vi "Write Result.vi"(8 "error in (no error)":errorcluster, 11 "TestData":T1 {"data"."Settings"."Source V" format="%#_g V"; "data"."Settings"."VLED 3" format="%#_g V"; "data"."Settings"."VLED 2" format="%#_g V"; "data"."Settings"."VLED 1" format="%#f V"; "data"."Limits"."Wavelength" format="%#_g nm"; "data"."Limits"."Tolerance" format="%#_g %"; "data"."Limits"."Current 3" format="%#_g  mA"; "data"."Limits"."Current 2" format="%#_g  mA"; "data"."Limits"."Current 1" format="%#_g mA"; "data"."Instruments"."Resistor 3" format="%#_g ohm"; "data"."Instruments"."Resistor 2" format="%#_g ohm"; "data"."Instruments"."Resistor 1" format="%#f ohm"}) -> (0 "error out":errorcluster, 2 "History Data":string[](array[string]))   [LabVIEW 2018, in "LED Control Module.lvlib"]
doc: "Very simple result logger - this is a placeholder."
uses:
  LED Control Module.lvlib
  Public Controls/TestData.ctl
  INI/INI File Control.ctl
  Public Controls/LVS Testplan.ctl
  Public Controls/LVS Instruments.ctl
  Public Controls/LVS Limits.ctl
  Public Controls/LVS Settings.ctl
  <vilib>/Utility/file.llb/Write Delimited Spreadsheet (string).vi
  INI/LED INI File.lvlib
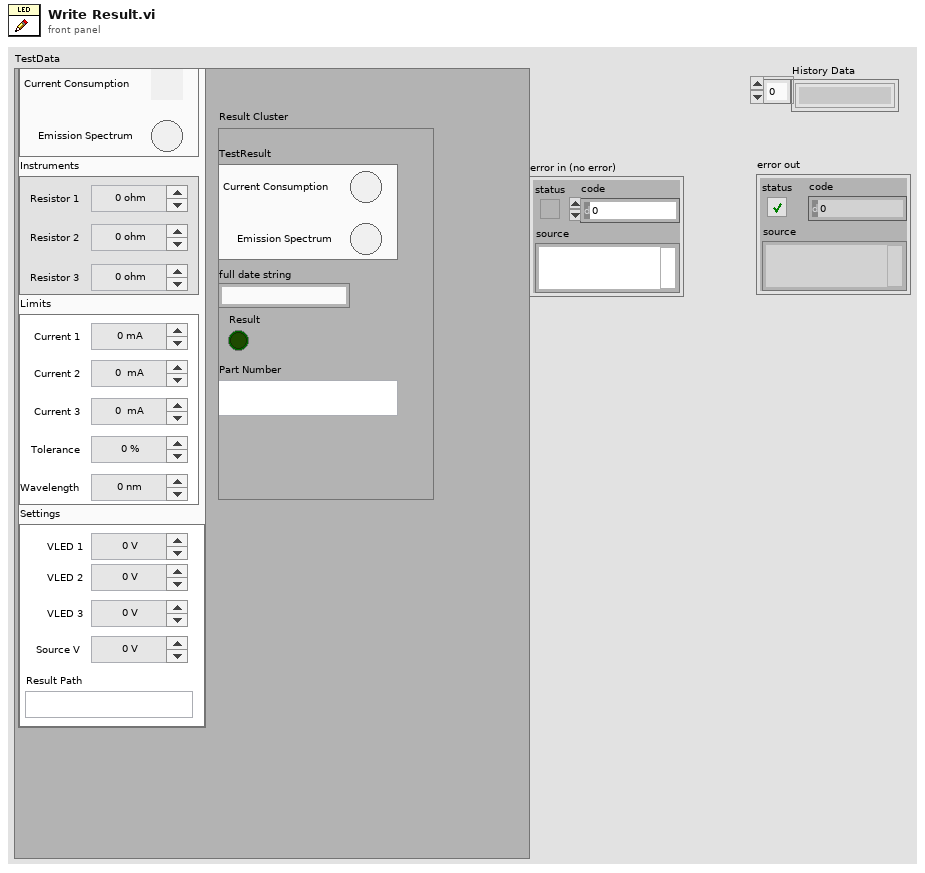
[diagram p1: front panel]
types:
  T1 = typedef "LED Control Module.lvlib/TestData.ctl" = cluster{"data":T2, "Result Cluster":cluster{"TestResult":T3, "full date string":string, "Result":bool, "Part Number":string}}
  T2 = typedef "LED Control Module.lvlib/LED INI File.lvlib/INI File Control.ctl" = cluster{"TestPlan":T3, "Instruments":T4, "Limits":T5, "Settings":T6}
  T3 = typedef "LED Control Module.lvlib/LVS Testplan.ctl" = cluster{"Current Consumption":bool, "Emission Spectrum":bool}
  T4 = typedef "LED Control Module.lvlib/LVS Instruments.ctl" = cluster{"Resistor 1":dbl, "Resistor 2":dbl, "Resistor 3":dbl}
  T5 = typedef "LED Control Module.lvlib/LVS Limits.ctl" = cluster{"Current 1":dbl, "Current 2":dbl, "Current 3":dbl, "Tolerance":dbl, "Wavelength":dbl}
  T6 = typedef "LED Control Module.lvlib/LVS Settings.ctl" = cluster{"VLED 1":dbl, "VLED 2":dbl, "VLED 3":dbl, "Source V":dbl, "Result Path":path}
  T7 = enum16{"open", "replace", "create", "open or create", "replace or create", "replace or create with confirmation"}
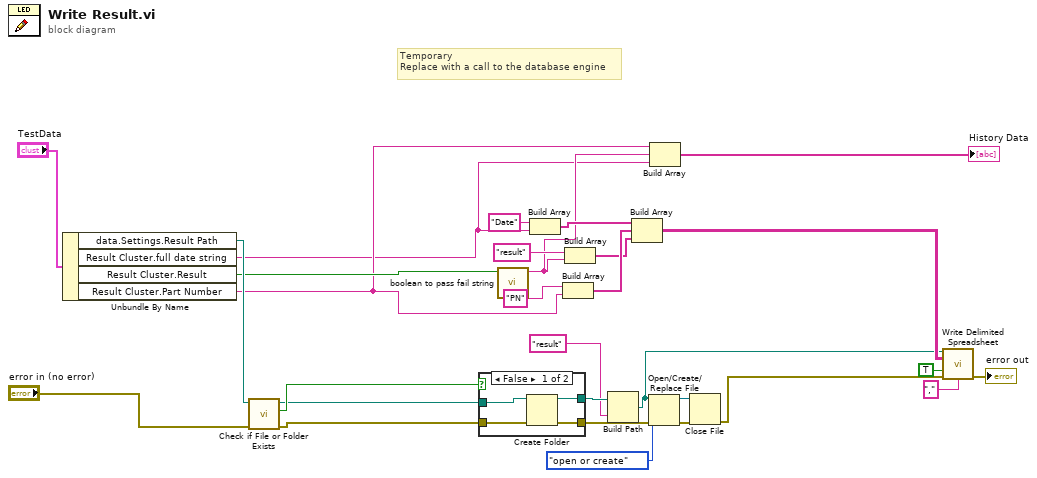
[diagram p0: block diagram]
diagram:
  # "Temporary\nReplace with a call to the database engine"
  n1 = Unbundle By Name("TestData") -> ("data.Settings.Result Path"=w28:path, "Result Cluster.full date string"=w2:string, "Result Cluster.Result"=w20:bool, "Result Cluster.Part Number"=w4:string)
  n2 = call <vilib>:"Check if File or Folder Exists.vi"("error in (no error)"="error in (no error)", "path"=w28) -> ("error out"=w25:errorcluster, "file or folder exists?"=w27:bool, "dup path"=w26:path)  [unwired: 7 in]
  n3 = case shown="False" w27 {
    tunnel: w26 -> [w33 w35]
    tunnel: w25 -> [w32 w34]
    tunnel: [w31 w34] -> w23
    tunnel: [w30 w35] -> w12
    frame False {
      n4 = Create Folder(path (use dialog)=w33, error in=w32) -> (created path=w30:path, error out=w31:errorcluster)  [unwired: 1 in, 1 out]
    }
    frame True {
    }
  }
  n5 = call "boolean to pass fail string.vi"("Boolean"=w20) -> ("Stat"=w3:string)  [unwired: 9 in, 1 out]
  n6 = Build Array("Date" ("element"), w2) -> (w18:string[])
  n7 = Build Array("PN" ("element"), w4) -> (w6:string[])
  n8 = Build Array("result" ("element"), w3) -> (w5:string[])
  n9 = Build Path(base path=w12, name or relative path="result") -> (appended path=w10:path)
  n10 = Build Array(w18, w6, w5) -> (w17:string[][])
  n11 = Open/Create/Replace File(file path (use dialog)=w10, error in=w23, operation (0:open)=T7."open or create") -> (refnum out=w14:refnum<file>, error out=w15:errorcluster)  [unwired: 3 in, 1 out]
  n12 = Build Array(w4, w3, w2) -> (→"History Data":string[])
  n13 = Close File(refnum=w14, error in=w15) -> (error out=w13:errorcluster)  [unwired: 1 out]
  n14 = call-poly <vilib>:"Write Delimited Spreadsheet.vi"("file path (dialog if empty)"=w10, "2D data"=w17, "append to file? (new file:F)"=TRUE, "error in (no error)"=w13, "delimiter (\\t)"="," ("delimiter (\\t)")) -> ("error out"=→"error out":errorcluster)  [unwired: 9 in, 1 out]
